vi "Shoot.vi"(1 "Shoot":bool, 2 "Aiming":bool) -> (0 "Done":bool)   [LabVIEW 2013]
uses:
  Robot Global Data.vi
panel:
  in  "Rest Position 2":dbl=51.0
  in  "Load Position 2":dbl=115.0
  in  "Pause Duration":u32=500
  out "Pause Start Time":i32=3072743
  out "Pausing":bool
  in  "Gate Duration":u32=150
  out "Gate Start Time":i32=3072170
  out "Gate Opening":bool
  in  "Shoot Duration":u32=400
  in  "Rest Position 1":dbl=80.0
  out "Shoot Start Time":i32=3072321
  in  "Load Position 1":dbl=170.0
  out "Shooting":bool
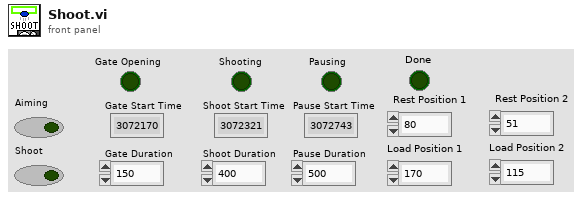
[diagram p1: front panel]
types:
  T1 = cluster{"Gate Opening":bool, "Shooting":bool, "Pausing":bool}
  T2 = typedef "WPI_ServoDeviceRef.ctl" = cluster{"DeviceStatus":errorcluster, "Digital Module":T3, "PWM Channel":T4, "DeadBand":T5}
  T3 = typedef "FPGA_TypedefDigitalModule.ctl" = enum16{"Digital Module 1", "Digital Module 2"}
  T4 = typedef "FPGA_DIOPWMChannel.ctl" = enum8{"PWM 1", "PWM 2", "PWM 3", "PWM 4", "PWM 5", "PWM 6", "PWM 7", "PWM 8", "PWM 9", "PWM 10", "Invalid"}
  T5 = typedef "WPI_PWMDeadband.ctl" = cluster{"Name":string, "maxPositivePwm":i32, "minPositivePwm":i32, "centerPwm":i32, "maxNegativePwm":i32, "minNegativePwm":i32, "angularRange":u16}
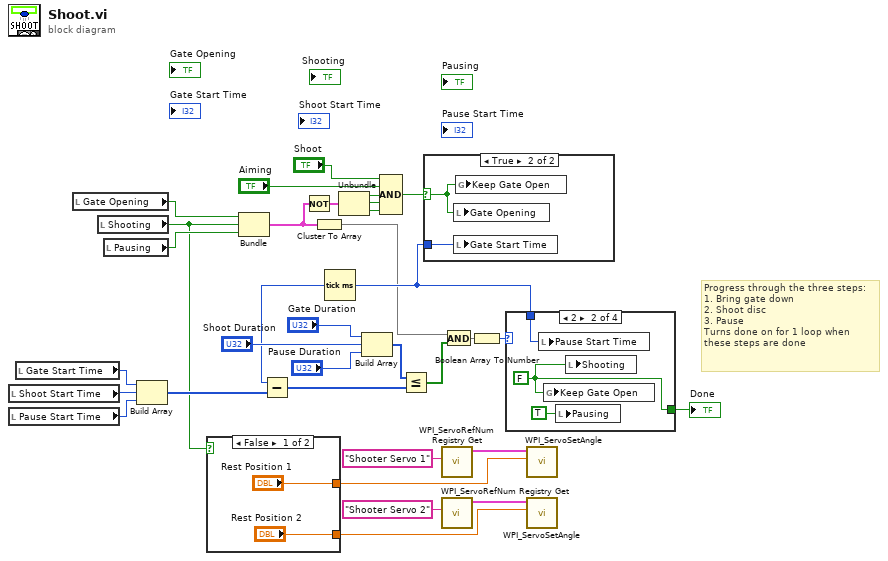
[diagram p0: block diagram]
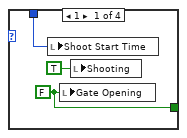
[diagram p2: hidden frame]
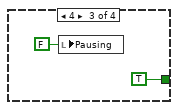
[diagram p3: hidden frame]
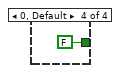
[diagram p4: hidden frame]
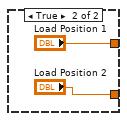
[diagram p6: hidden frame]
diagram:
  # "Progress through the three steps:\n1. Bring gate down\n2. Shoot disc\n3. Pause\nTurns done on for 1 loop when\nthese steps are done"
  n1 = local read "Shoot Start Time"() -> (w26:i32)
  n2 = local read "Pause Start Time"() -> (w25:i32)
  n3 = local read "Gate Start Time"() -> (w27:i32)
  n4 = local read "Gate Opening"() -> (w14:bool)
  n5 = local read "Shooting"() -> (w6:bool)
  n6 = local read "Pausing"() -> (w13:bool)
  n7 = Build Array(w27, w26, w25) -> (w24:i32[])
  n8 = case shown="False" w6 {
    tunnel: ["Rest Position 1" "Load Position 1"] -> w3
    tunnel: ["Rest Position 2" "Load Position 2"] -> w1
    frame False {
    }
    frame True {
    }
  }
  n9 = Bundle("Gate Opening"=w14, "Shooting"=w6, "Pausing"=w13) -> (w11:T1)  [unwired: 1 in]
  n10 = Not(x=w11) -> (.not. x?=w10:T1)
  n11 = Cluster To Array(cluster=w11) -> (array=w12:bool[])
  n12 = Tick Count (ms)() -> (millisecond timer value=w16:u32)
  n13 = Subtract(x=w16, y=w24) -> (x-y=w19:u32[])
  n14 = Unbundle(w10) -> ("Gate Opening"=w9:bool, "Shooting"=w8:bool, "Pausing"=w7:bool)
  n15 = Build Array("Gate Duration", "Shoot Duration", "Pause Duration") -> (w20:u32[])
  n16 = Compound Arithmetic op=AND("Shoot", "Aiming", w9, w8, w7) -> (w29:bool)
  n17 = Less Or Equal?(x=w20, y=w19) -> (x <= y?=w18:bool[])
  n18 = case shown="True" w29 {
    selector: w29 -> [_ w37]
    tunnel: w16 -> [_ w38]
    frame False {
    }
    frame True {
      n19 = local write "Gate Opening"(w37) -> ()
      n20 = local write "Gate Start Time"(w38) -> ()
      n21 = global write "Robot Global Data.vi" "Keep Gate Open"(w37) -> ()
    }
  }
  n22 = call <vilib>:"WPI_ServoRefNum Registry Get.vi"("refnum name"="Shooter Servo 1") -> ("ServoDeviceRef"=w31:T2)  [unwired: 9 in, 1 out]
  n23 = call <vilib>:"WPI_ServoRefNum Registry Get.vi"("refnum name"="Shooter Servo 2") -> ("ServoDeviceRef"=w2:T2)  [unwired: 9 in, 1 out]
  n24 = And(x=w12, y=w18) -> (x .and. y?=w15:bool[])
  n25 = Boolean Array To Number(Boolean array=w15) -> (number=w17:u32)
  n26 = case shown="2" w17 {
    tunnel: w16 -> [w40 w44 _ _]
    tunnel: [w39 w42 TRUE FALSE] -> w5
    frame 1 {
      w39 = FALSE ("Gate Opening")
      n27 = local write "Shoot Start Time"(w40) -> ()
      n28 = local write "Gate Opening"(w39) -> ()
      n29 = local write "Shooting"(TRUE ("Shooting")) -> ()
    }
    frame 2 {
      w42 = FALSE ("Keep Gate Open")
      n30 = local write "Pause Start Time"(w44) -> ()
      n31 = global write "Robot Global Data.vi" "Keep Gate Open"(w42) -> ()
      n32 = local write "Pausing"(TRUE ("Pausing")) -> ()
      n33 = local write "Shooting"(w42) -> ()
    }
    frame 4 {
      n34 = local write "Pausing"(FALSE ("Pausing")) -> ()
    }
    frame 0, Default {
    }
  }
  "Done" <- w5
  n35 = call <vilib>:"WPI_ServoSetAngle.vi"("Angle"=w3, "ServoDeviceRef"=w31) -> ()  [unwired: 8 in, 2 out]
  n36 = call <vilib>:"WPI_ServoSetAngle.vi"("Angle"=w1, "ServoDeviceRef"=w2) -> ()  [unwired: 8 in, 2 out]
